vi "Bind Terminal.vi"(7 "Use Label Text (F=Use Caption)":bool, 8 "error in (no error)":errorcluster, 9 "Topic Name (Use Control Text)":string, 10 "Ctl Refnum":refnum<vi>, 11 "IObserver in":refnum<class "IObserver.lvclass">) -> (0 "error out":errorcluster, 3 "IObserver out":refnum<class "IObserver.lvclass">)   [LabVIEW 2015, in "IObserver.lvlib" / "IObserver.lvclass"]
uses:
  IObserver.lvclass
  <vilib>/ActorFramework/Actor/Actor.lvclass/Actor.ctl
  <vilib>/ActorFramework/Message Enqueuer/Message Enqueuer.lvclass/Message Enqueuer.ctl
  IObserver Messages/Subscribe Msg/Subscribe Msg.lvclass/Subscribe Msg.ctl
  <vilib>/ActorFramework/Message Enqueuer/Init from Existing Queue.vi
  <vilib>/ActorFramework/Message Enqueuer/Enqueue.vi
  <vilib>/ActorFramework/Message Priority Queue/Priority Enqueue.vi
  <vilib>/ActorFramework/Message Enqueuer/Message Enqueuer.lvclass
  IObserver Messages/Subscribe Msg/Subscribe Msg.lvclass
  IMediator/SubscriptionRequest/SubscriptionRequest.lvclass
  <vilib>/ActorFramework/Actor/Actor.lvclass
  Mediator/Transport/TerminalBinding/TerminalBinding.lvclass
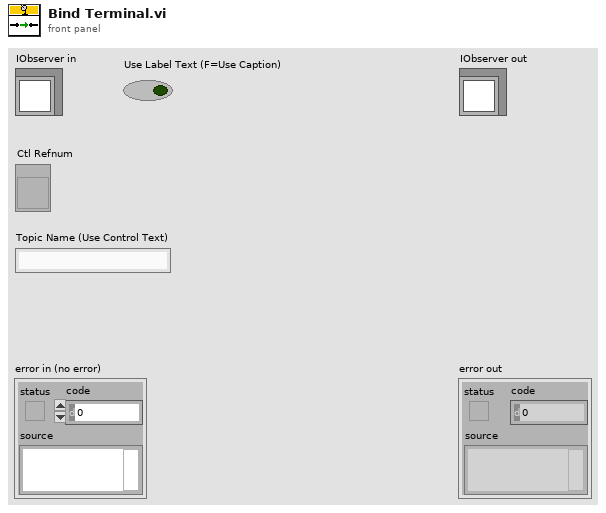
[diagram p1: front panel]
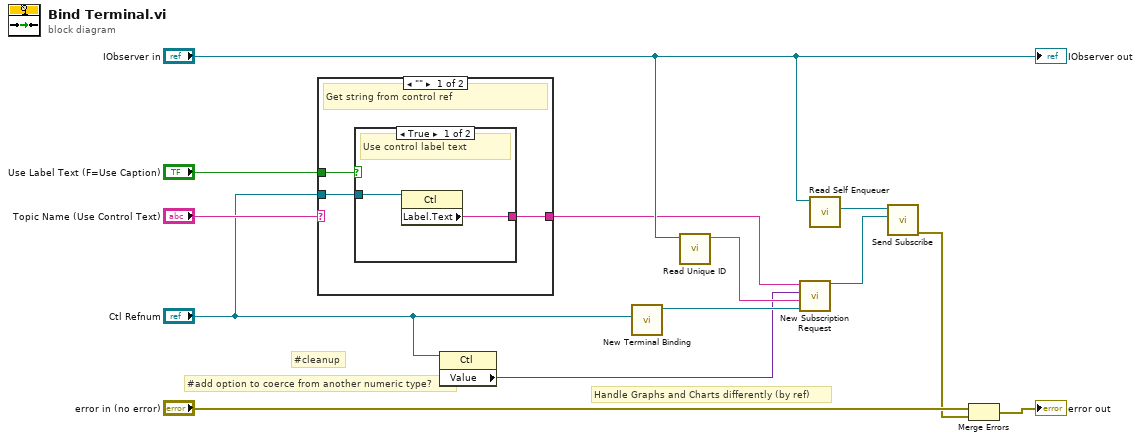
[diagram p0: block diagram]
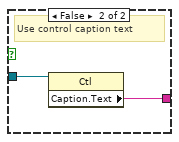
[diagram p2: hidden frame]
diagram:
  # "Handle Graphs and Charts differently (by ref)"
  # "#add option to coerce from another numeric type?"
  # "#cleanup"
  n1 = case shown="\"\"" "Topic Name (Use Control Text)" {
    selector: "Topic Name (Use Control Text)" -> [_ w21]
    tunnel: [w14 w21] -> w2
    tunnel: "Use Label Text (F=Use Caption)" -> [w16 _]
    tunnel: "Ctl Refnum" -> [w15 _]
    frame "" {
      # "Get string from control ref"
      n2 = case shown="True" w16 {
        tunnel: w15 -> [w18 w20]
        tunnel: [w17 w19] -> w14
        frame True {
          # "Use control label text"
          n3 = property class="Ctl"(reference=w18) -> ("Label.Text"=w17:string)  [unwired: 1 in, 2 out]
        }
        frame False {
          # "Use control caption text"
          n4 = property class="Ctl"(reference=w20) -> ("Caption.Text"=w19:string)  [unwired: 1 in, 2 out]
        }
      }
    }
    frame Default {
      # "Use string wired to input terminal"
    }
  }
  n5 = property class="Ctl"(reference="Ctl Refnum") -> ("Value"=w10:variant)  [unwired: 1 in, 2 out]
  n6 = call "New Terminal Binding.vi"("Ctl Refnum"="Ctl Refnum") -> ("TerminalBinding out"=w12:refnum<class "TerminalBinding.lvclass">)  [unwired: 9 in, 1 out]
  n7 = call "Read Unique ID.vi"("IObserver In"="IObserver in") -> ("Unique ID"=w11:string)  [unwired: 10 in]
  n8 = call "New Subscription Request.vi"("Transport"=w12, "Unique Subscriber ID"=w11, "Type"=w10, "Topic Name"=w2) -> ("SubscriptionRequest out"=w7:refnum<class "SubscriptionRequest.lvclass">)  [unwired: 7 in]
  n9 = call <vilib>:"Read Self Enqueuer.vi"("Actor"="IObserver in") -> ("Self Enqueuer"=w8:refnum<class "Message Enqueuer.lvclass">)  [unwired: 10 in]
  n10 = call "Send Subscribe.vi"("SubscriptionRequest"=w7, "Message Enqueuer"=w8) -> ("error out"=w5:errorcluster)  [unwired: 8 in, 1 out]
  n11 = Merge Errors("error in (no error)", w5) -> (→"error out":errorcluster)
  "IObserver out" <- "IObserver in"
